vi "Write IV_data.lvclass.vi"(8 "error in (no error)":errorcluster, 10 "IV_data.lvclass":refnum<class "IV_data.lvclass">, 11 "IV in":refnum<class "IV.lvclass">) -> (0 "error out":errorcluster, 3 "IV out":refnum<class "IV.lvclass">)   [LabVIEW 2014, in "IV.lvclass"]
uses:
  IV.lvclass
  data/IV_data.lvclass
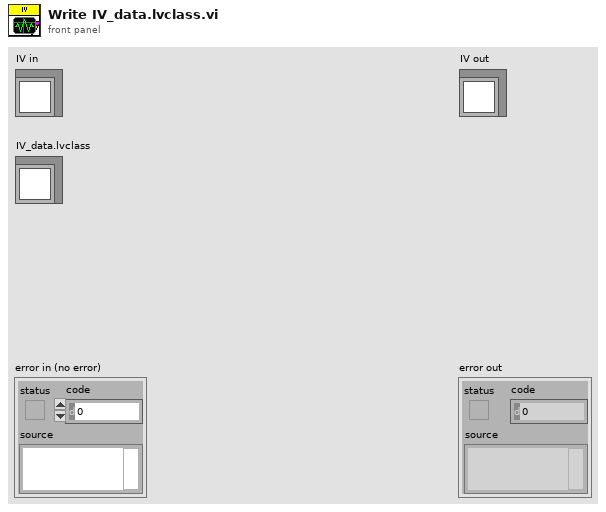
[diagram p1: front panel]
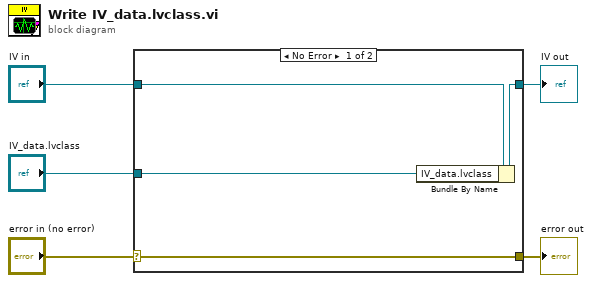
[diagram p0: block diagram]
diagram:
  n1 = case shown="No Error" "error in (no error)" {
    selector: "error in (no error)" -> [w9 w10]
    tunnel: [w9 w10] -> w4
    tunnel: [w7 w11] -> w2
    tunnel: "IV in" -> [w8 w11]
    tunnel: "IV_data.lvclass" -> [w6 _]
    frame No Error {
      n2 = Bundle By Name(cluster=w8, "IV_data.lvclass"=w6) -> (w7:refnum<class "IV.lvclass">)
    }
    frame Error {
    }
  }
  "error out" <- w4
  "IV out" <- w2
